vi "FixAngle.vi"(11 "Angle To Turn in":dbl) -> (3 "Angle To Turn out":dbl)   [LabVIEW 2015]
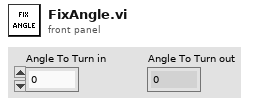
[diagram p1: front panel]
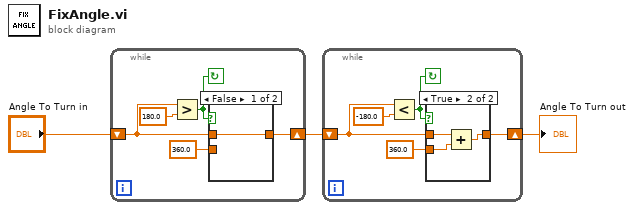
[diagram p0: block diagram]
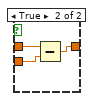
[diagram p3: hidden frame]
diagram:
  n1 = while {
    shift-right: [w5] -> w2
    shift-left: "Angle To Turn in" -> [w6]
    stop <- w7 continue-if-true
    n2 = Greater?(x=w6, y=180.0) -> (0:w7:bool)
    n3 = case shown="False" w7 {
      tunnel: w6 -> [w9 w12]
      tunnel: 360.0 -> [_ w11]
      tunnel: [w9 w10] -> w5
      frame False {
      }
      frame True {
        n4 = Subtract(x=w12, y=w11) -> (x-y=w10:dbl)
      }
    }
  }
  n5 = while {
    shift-right: [w14] -> w1
    shift-left: w2 -> [w15]
    stop <- w16 continue-if-true
    n6 = Less?(x=w15, y=-180.0) -> (x < y?=w16:bool)
    n7 = case shown="True" w16 {
      tunnel: w15 -> [w18 w21]
      tunnel: 360.0 -> [_ w20]
      tunnel: [w18 w19] -> w14
      frame False {
      }
      frame True {
        n8 = Add(x=w21, y=w20) -> (x+y=w19:dbl)
      }
    }
  }
  "Angle To Turn out" <- w1
